vi "Flock_Master_WriteNewRev.vi"(0 "configuration file path":path=path "C:/Users/mblack/test/mblack-harrypotter2-test/user/mblack/FRC Team Service/Trunk/2.0/Master/source/Static Source/master/FRCts.ini", 1 "MajorRev":i32=2, 2 "MinorRev":i32, 3 "BuildPhase":string="a", 4 "BuildNum":i32, 5 "error in (no error)":errorcluster, 6 "BranchNum":i32) -> (19 "error out":errorcluster)   [LabVIEW 2013, in "Flock_Master_BuildRevision.lvlib"]
uses:
  Flock_Master_BuildRevision.lvlib
  <vilib>/Utility/config.llb/Write Key (I32).vi
  <vilib>/Utility/config.llb/Write Key (String).vi
  <vilib>/Utility/config.llb/NI_LVConfig.lvlib
panel:
  in  "create file if necessary (T)":bool=TRUE
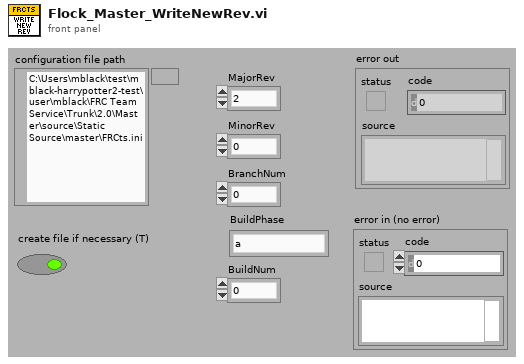
[diagram p1: front panel]
types:
  T1 = typedef "NI_LVConfig.lvlib/Config Data RefNum.ctl" = refnum<k1>
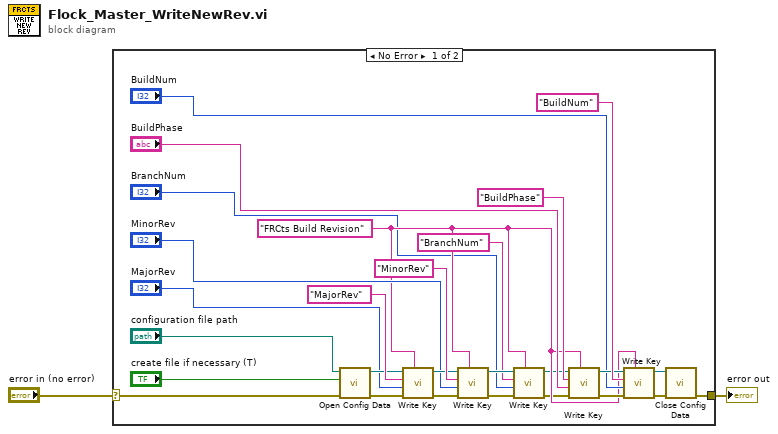
[diagram p0: block diagram]
diagram:
  n1 = case shown="No Error" "error in (no error)" {
    selector: "error in (no error)" -> [w10 w30]
    tunnel: [w12 w30] -> w2
    frame No Error {
      w8 = "FRCts Build Revision"
      n2 = call <vilib>:"Open Config Data.vi"("error in (no error)"=w10, "create file if necessary (T)"="create file if necessary (T)", "configuration file path"="configuration file path") -> ("error out"=w21:errorcluster, "refnum"=w20:T1)  [unwired: 6 in, 1 out]
      n3 = call-poly <vilib>:"Write Key.vi"("section"=w8, "error in (no error)"=w21, "value"="MajorRev", "key"="MajorRev", "refnum"=w20) -> ("error out"=w24:errorcluster, "refnum out"=w23:T1)  [unwired: 4 in, 1 out]
      n4 = call-poly <vilib>:"Write Key.vi"("section"=w8, "error in (no error)"=w24, "value"="MinorRev", "key"="MinorRev", "refnum"=w23) -> ("error out"=w7:errorcluster, "refnum out"=w9:T1)  [unwired: 4 in, 1 out]
      n5 = call-poly <vilib>:"Write Key.vi"("section"=w8, "error in (no error)"=w7, "value"="BranchNum", "key"="BranchNum", "refnum"=w9) -> ("error out"=w6:errorcluster, "refnum out"=w3:T1)  [unwired: 4 in, 1 out]
      n6 = call-poly <vilib>:"Write Key.vi"("section"=w8, "error in (no error)"=w6, "value"="BuildPhase", "key"="BuildPhase", "refnum"=w3) -> ("error out"=w27:errorcluster, "refnum out"=w28:T1)  [unwired: 4 in, 1 out]
      n7 = call-poly <vilib>:"Write Key.vi"("section"=w8, "error in (no error)"=w27, "value"="BuildNum", "key"="BuildNum", "refnum"=w28) -> ("error out"=w13:errorcluster, "refnum out"=w11:T1)  [unwired: 4 in, 1 out]
      n8 = call <vilib>:"Close Config Data.vi"("error in (no error)"=w13, "refnum"=w11) -> ("error out"=w12:errorcluster)  [unwired: 8 in, 1 out]
    }
    frame Error {
    }
  }
  "error out" <- w2
